vi "统计全局变量.vi"() -> ()   [LabVIEW 2016]
panel:
  in  "实际备注数组":string[](array[string])
  in  "历史数据":sgl[][](array[numeric])
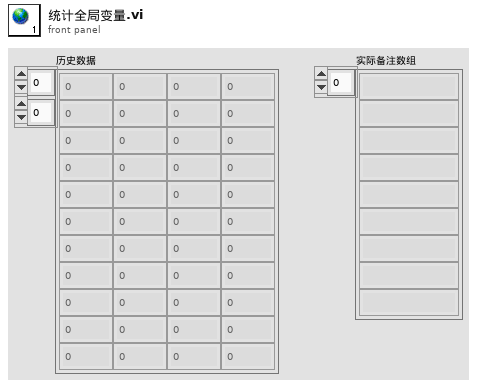
[diagram p1: front panel]
diagram:
